vi "Init Robot.vi"(0 "Brake 35":bool=TRUE, 1 "Brake 40":bool=TRUE, 4 "Brake Switch 40":bool=TRUE, 5 "Brake Switch 35":bool=TRUE, 6 "Left Pot Gradient":dbl, 7 "Right Pot Gradient":dbl, 8 "Left Pot Offset":dbl, 9 "Right Pot Offset":dbl) -> (12 "Left Pot Init Reading":dbl, 13 "Right Pot Init Reading":dbl, 14 "Force bias LX":dbl, 15 "Force bias LY":dbl, 16 "Force bias RX":dbl, 17 "Force bias RY":dbl, 18 "Initial Translation":dbl, 19 "Initial Rotation":dbl)   [LabVIEW 2019]
uses:
  <vilib>/myRIO/Instrument Drivers/Onboard IO/AO/typedefs/AO Reference.ctl
  <vilib>/myRIO/Common/Instrument Driver Framework/Utilities/typedefs/myRIO Generic Hardware Reference.ctl
  <vilib>/myRIO/Common/Instrument Driver Framework/Utilities/typedefs/Hardware Version Enum.ctl
  <vilib>/myRIO/Common/Instrument Driver Framework/Utilities/typedefs/myRIO v1.0 Reference.ctl
  <vilib>/myRIO/Common/Instrument Driver Framework/Utilities/typedefs/Generic FPGA Reference.ctl
  <vilib>/myRIO/Common/Instrument Driver Framework/myRIO v1.0/AO/typedefs/AO Channels List.ctl
  <vilib>/myRIO/Common/Instrument Driver Framework/myRIO v1.0/AO/typedefs/AO Channels Enum.ctl
  <vilib>/myRIO/Common/Instrument Driver Framework/Utilities/typedefs/Analog Scaling Constants List.ctl
  <vilib>/myRIO/Common/Instrument Driver Framework/Utilities/typedefs/Analog Scaling Constants.ctl
  <vilib>/userDefined/High Color/nirio_resource_hc.ctl
  <vilib>/myRIO/Instrument Drivers/Onboard IO/DIO/typedefs/DIO Reference.ctl
  <vilib>/myRIO/Common/Instrument Driver Framework/myRIO v1.0/DIO/typedefs/DIO Channels List.ctl
  <vilib>/myRIO/Common/Instrument Driver Framework/myRIO v1.0/DIO/typedefs/DIO Channels Enum.ctl
  <vilib>/myRIO/Instrument Drivers/Onboard IO/AI/typedefs/AI Reference.ctl
  <vilib>/myRIO/Common/Instrument Driver Framework/myRIO v1.0/AI/typedefs/AI Channels List.ctl
  <vilib>/myRIO/Common/Instrument Driver Framework/myRIO v1.0/AI/typedefs/AI Channels Enum.ctl
  <vilib>/myRIO/Common/Instrument Driver Framework/myRIO v1.0/Encoder/typedefs/Encoder Signal Mode.ctl
  <vilib>/myRIO/Instrument Drivers/Onboard IO/Encoder/typedefs/Encoder Reference.ctl
  <vilib>/myRIO/Common/Instrument Driver Framework/myRIO v1.0/Encoder/typedefs/Encoder Channels Enum.ctl
  <vilib>/myRIO/Common/Instrument Driver Framework/myRIO v1.0/Encoder/typedefs/Encoder Configuration v1.0.ctl
  <vilib>/myRIO/Common/Instrument Driver Framework/Utilities/vis/Is FPGA Ref Available.vi
  <vilib>/myRIO/Common/Instrument Driver Framework/myRIO v1.0/AO/vis/myRIO v1.1 Open AO.vi
  <vilib>/myRIO/Instrument Drivers/Onboard IO/AO/vis/Write.vi
  <vilib>/myRIO/Common/Instrument Driver Framework/myRIO v1.0/DIO/vis/myRIO v1.1 Open DIO.vi
  <vilib>/myRIO/Instrument Drivers/Onboard IO/DIO/vis/Write.vi
  <vilib>/myRIO/Common/Instrument Driver Framework/myRIO v1.0/AI/vis/myRIO v1.1 Open AI.vi
  <vilib>/myRIO/Instrument Drivers/Onboard IO/AI/vis/Read.vi
  <vilib>/myRIO/Common/Instrument Driver Framework/myRIO v1.0/Encoder/vis/myRIO v1.1 Open Encoder.vi
  <vilib>/myRIO/Instrument Drivers/Onboard IO/Encoder/vis/Read.vi
  <vilib>/myRIO/Common/Instrument Driver Framework/Utilities/vis/Validate Channels.vi
  <vilib>/myRIO/Common/Instrument Driver Framework/myRIO v1.0/AO/vis/myRIO v1.0 Reserve AO.vi
  <vilib>/myRIO/Common/Instrument Driver Framework/myRIO v1.0/DIO/vis/myRIO v1.0 Reserve DIO.vi
  <vilib>/myRIO/Common/Instrument Driver Framework/myRIO v1.0/AI/vis/myRIO v1.0 Reserve AI.vi
  <vilib>/myRIO/Common/Instrument Driver Framework/myRIO v1.0/Encoder/vis/myRIO v1.0 Reserve Encoder.vi
  <vilib>/myRIO/Common/Instrument Driver Framework/myRIO v1.0/AO/vis/myRIO v1.0 Build MUX Configuration AO.vi
  <vilib>/myRIO/Common/Instrument Driver Framework/myRIO v1.0/Resource Manager/vis/myRIO v1.0 Reserve Channel List.vi
  <vilib>/myRIO/Common/Instrument Driver Framework/myRIO v1.0/DIO/vis/myRIO v1.0 Build MUX Configuration DIO.vi
  <vilib>/myRIO/Common/Instrument Driver Framework/myRIO v1.0/AI/vis/myRIO v1.0 Build MUX Configuration AI.vi
  <vilib>/myRIO/Common/Instrument Driver Framework/myRIO v1.0/Encoder/vis/myRIO v1.0 Build MUX Configuration Encoder.vi
  <vilib>/myRIO/Common/Instrument Driver Framework/myRIO v1.0/Resource Manager/vis/myRIO v1.0 Reserve Channel.vi
  <vilib>/myRIO/Common/Instrument Driver Framework/myRIO v1.0/Resource Manager/vis/myRIO v1.0 Unreserve Channel.vi
  <vilib>/myRIO/Common/Instrument Driver Framework/myRIO v1.0/Resource Manager/vis/myRIO v1.0 Create Configuration List.vi
  <vilib>/myRIO/Common/Instrument Driver Framework/myRIO v1.0/Resource Manager/vis/myRIO v1.0 Build Mutex Name.vi
  <vilib>/Utility/VariantDataType/GetNumericInfo.vi
  <vilib>/Utility/error.llb/Error Cluster From Error Code.vi
  <vilib>/myRIO/Common/Instrument Driver Framework/myRIO v1.0/myRIO v1.1 Open.vi
  <vilib>/myRIO/Common/Instrument Driver Framework/myRIO v1.0/AO/vis/myRIO v1.0 Get Scaling Constants AO.vi
  <vilib>/myRIO/Common/Instrument Driver Framework/Utilities/vis/IO Manager.vi
  <vilib>/myRIO/Common/Instrument Driver Framework/Utilities/vis/Configuration Manager.vi
  <vilib>/myRIO/Common/Instrument Driver Framework/myRIO v1.0/myRIO v1.0 Close.vi
  <vilib>/myRIO/Common/Instrument Driver Framework/myRIO v1.0/AO/vis/myRIO v1.0 Write AO.vi
  <vilib>/myRIO/Common/Instrument Driver Framework/myRIO v1.0/Resource Manager/vis/myRIO v1.0 Configure IO.vi
  <vilib>/myRIO/Common/Instrument Driver Framework/myRIO v1.0/DIO/vis/myRIO v1.0 Write DIO.vi
  <vilib>/myRIO/Common/Instrument Driver Framework/myRIO v1.0/AI/vis/myRIO v1.0 Get Scaling Constants AI.vi
  <vilib>/myRIO/Common/Instrument Driver Framework/myRIO v1.0/AI/vis/myRIO v1.0 Read AI.vi
  <vilib>/myRIO/Common/Instrument Driver Framework/myRIO v1.0/Encoder/vis/myRIO v1.0 Configure Encoder.vi
  <vilib>/myRIO/Common/Instrument Driver Framework/myRIO v1.0/Encoder/vis/myRIO v1.0 Read Encoder.vi
  <vilib>/myRIO/Express VI/Onboard IO/AO/AO Express VI.xnode
  <vilib>/myRIO/Instrument Drivers/Onboard IO/AO/vis/myRIO AO Open.xnode
  <vilib>/myRIO/Express VI/Onboard IO/DO/DO Express VI.xnode
  <vilib>/myRIO/Instrument Drivers/Onboard IO/DIO/vis/myRIO DIO Open.xnode
  <vilib>/myRIO/Express VI/Onboard IO/AI/AI Express VI.xnode
  <vilib>/myRIO/Instrument Drivers/Onboard IO/AI/vis/myRIO AI Open.xnode
  <vilib>/myRIO/Express VI/Onboard IO/Encoder/Encoder Express VI.xnode
  <vilib>/myRIO/Instrument Drivers/Onboard IO/Encoder/vis/myRIO Encoder Open.xnode
  <vilib>/myRIO/Common/Instrument Driver Framework/myRIO v1.0/Encoder/typedefs/Encoder Count Direction Enum.ctl
  <vilib>/myRIO/Instrument Drivers/Onboard IO/Encoder/Encoder.lvlib
  <vilib>/myRIO/Instrument Drivers/Onboard IO/DIO/DIO.lvlib
  <vilib>/myRIO/Instrument Drivers/Onboard IO/AO/AO.lvlib
  <vilib>/myRIO/Instrument Drivers/Onboard IO/AI/AI.lvlib
panel:
  out "VoltageTranslation":dbl
  out "VoltageRotation":dbl
  out "Encoder Counter Value":i32(graph)
  out "Encoder Counter Value 2":i32(graph)
  out "P Rotation":dbl
  out "P Translation":dbl
  out "left init":dbl
  out "right init":dbl
  out "Rot Pot":dbl
  # "This Vi starts all task, calculates the initals values of all sensores and encoder and can open the brakes if needed."
  # "Output:"
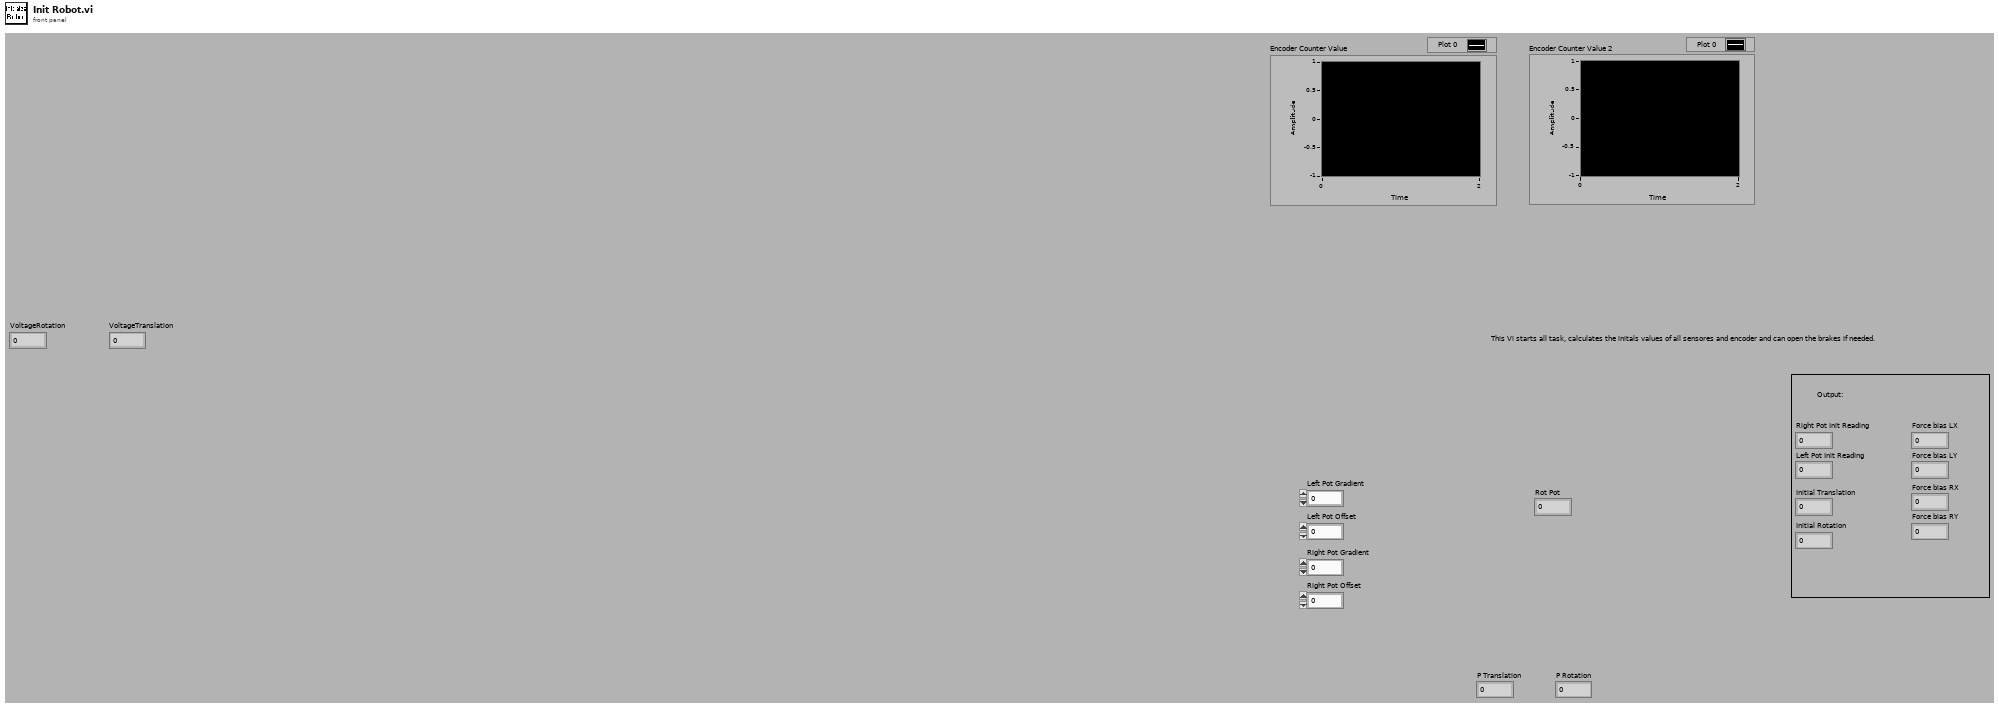
[diagram p1: front panel]
types:
  T1 = typedef "AO.lvlib/AO Reference.ctl" = cluster{"myRIO Reference":T2, "AO Channel List":T6, "AO Scaling Constant List":T8}
  T2 = typedef "myRIO Generic Hardware Reference.ctl" = cluster{"myRIO Model":T3, "myRIO Hardware Reference":T4}
  T3 = typedef "Hardware Version Enum.ctl" = enum16{"Unknown", "myRIO-1900", "myRIO-1950", "roboRIO", "NI ELVIS RIO CM", "ELVIS III"}
  T4 = typedef "myRIO v1.0 Reference.ctl" = cluster{"Generic FPGA Reference":T5, "Allow multiple opens":bool}
  T5 = typedef "Generic FPGA Reference.ctl" = refnum<k20>
  T6 = typedef "AO Channels List.ctl" = T7[]
  T7 = typedef "AO Channels Enum.ctl" = enum16{"Not Connected", "AudioOut/Left", "AudioOut/Right", "C/AO0", "C/AO1", "A/AO0", "A/AO1", "B/AO0", "B/AO1"}
  T8 = typedef "Analog Scaling Constants List.ctl" = T9[]
  T9 = typedef "Analog Scaling Constants.ctl" = cluster{"LSB Weight (Volts)":dbl, "Offset (Volts)":dbl, "Signed?":bool}
  T10 = typedef "nirio_resource_hc.ctl" = tag
  T11 = typedef "DIO.lvlib/DIO Reference.ctl" = cluster{"myRIO Reference":T2, "DIO Channels List":T12}
  T12 = typedef "DIO Channels List.ctl" = T13[]
  T13 = typedef "DIO Channels Enum.ctl" = enum16{"Not Connected", "C/DIO0", "C/DIO1", "C/DIO2", "C/DIO3", "C/DIO4", "C/DIO5", "C/DIO6", "C/DIO7", "A/DIO0", "A/DIO1", "A/DIO2", "A/DIO3", "A/DIO4", "A/DIO5", "A/DIO6", "A/DIO7", "A/DIO8", "A/DIO9", "A/DIO10", "A/DIO11", "A/DIO12", "A/DIO13", "A/DIO14", "A/DIO15", "A/DIO16", "A/DIO17", "A/DIO18", "A/DIO19", "B/DIO0", "B/DIO1", "B/DIO2", "B/DIO3", "B/DIO4", "B/DIO5", "B/DIO6", "B/DIO7", "B/DIO8", "B/DIO9", "B/DIO10", "B/DIO11", "B/DIO12", "B/DIO13", "B/DIO14", "B/DIO15", "B/DIO16", "B/DIO17", "B/DIO18", "B/DIO19", "LED0", "LED1", "LED2", "LED3", "Button0", "DIO/DIO0", "DIO/DIO1", "DIO/DIO2", "DIO/DIO3", "DIO/DIO4", "DIO/DIO5", "DIO/DIO6", "DIO/DIO7", "DIO/DIO8", "DIO/DIO9", "SPI/CS0", "SPI/CS1", "SPI/CS2", "SPI/CS3", "LED RADIO (Green)", "LED RADIO (Red)", "LED COMM (Green)", "LED COMM (Red)", "LED MODE (Green)", "LED MODE (Red)"}
  T14 = typedef "AI.lvlib/AI Reference.ctl" = cluster{"myRIO Reference":T2, "AI Channels List":T15, "AI Scaling Constants List":T8}
  T15 = typedef "AI Channels List.ctl" = T16[]
  T16 = typedef "AI Channels Enum.ctl" = enum16{"Not Connected", "AudioIn/Left", "AudioIn/Right", "C/AI0", "C/AI1", "A/AI0", "A/AI1", "A/AI2", "A/AI3", "A/AI4", "A/AI5", "A/AI6", "A/AI7", "B/AI0", "B/AI1", "B/AI2", "B/AI3", "B/AI4", "B/AI5", "B/AI6", "B/AI7", "AI/AI0", "AI/AI1", "AI/AI2", "AI/AI3", "A/AI0 (DIFF)", "A/AI1 (DIFF)", "A/AI2 (DIFF)", "A/AI3 (DIFF)", "B/AI0 (DIFF)", "B/AI1 (DIFF)", "B/AI2 (DIFF)", "B/AI3 (DIFF)"}
  T17 = typedef "Encoder.lvlib/Encoder Reference.ctl" = cluster{"myRIO Reference":T2, "Encoder Channels Enum":T18}
  T18 = typedef "Encoder Channels Enum.ctl" = enum16{"Not Connected", "C/ENC0", "C/ENC1", "A/ENC", "A/ENC0", "A/ENC1", "A/ENC2", "A/ENC3", "A/ENC4", "A/ENC5", "A/ENC6", "A/ENC7", "A/ENC8", "A/ENC9", "B/ENC", "B/ENC0", "B/ENC1", "B/ENC2", "B/ENC3", "B/ENC4", "B/ENC5", "B/ENC6", "B/ENC7", "B/ENC8", "B/ENC9", "DIO/ENC0", "DIO/ENC1", "DIO/ENC2", "DIO/ENC3", "DIO/ENC4"}
  T19 = typedef "Encoder Signal Mode.ctl" = enum16{"Quadrature phase signal", "Step and direction signal"}
  T20 = cluster{"[0]":dbl, "[1]":dbl, "[2]":dbl, "[3]":dbl, "[4]":dbl, "[5]":dbl, "[6]":dbl, "[7]":dbl, "[8]":dbl}
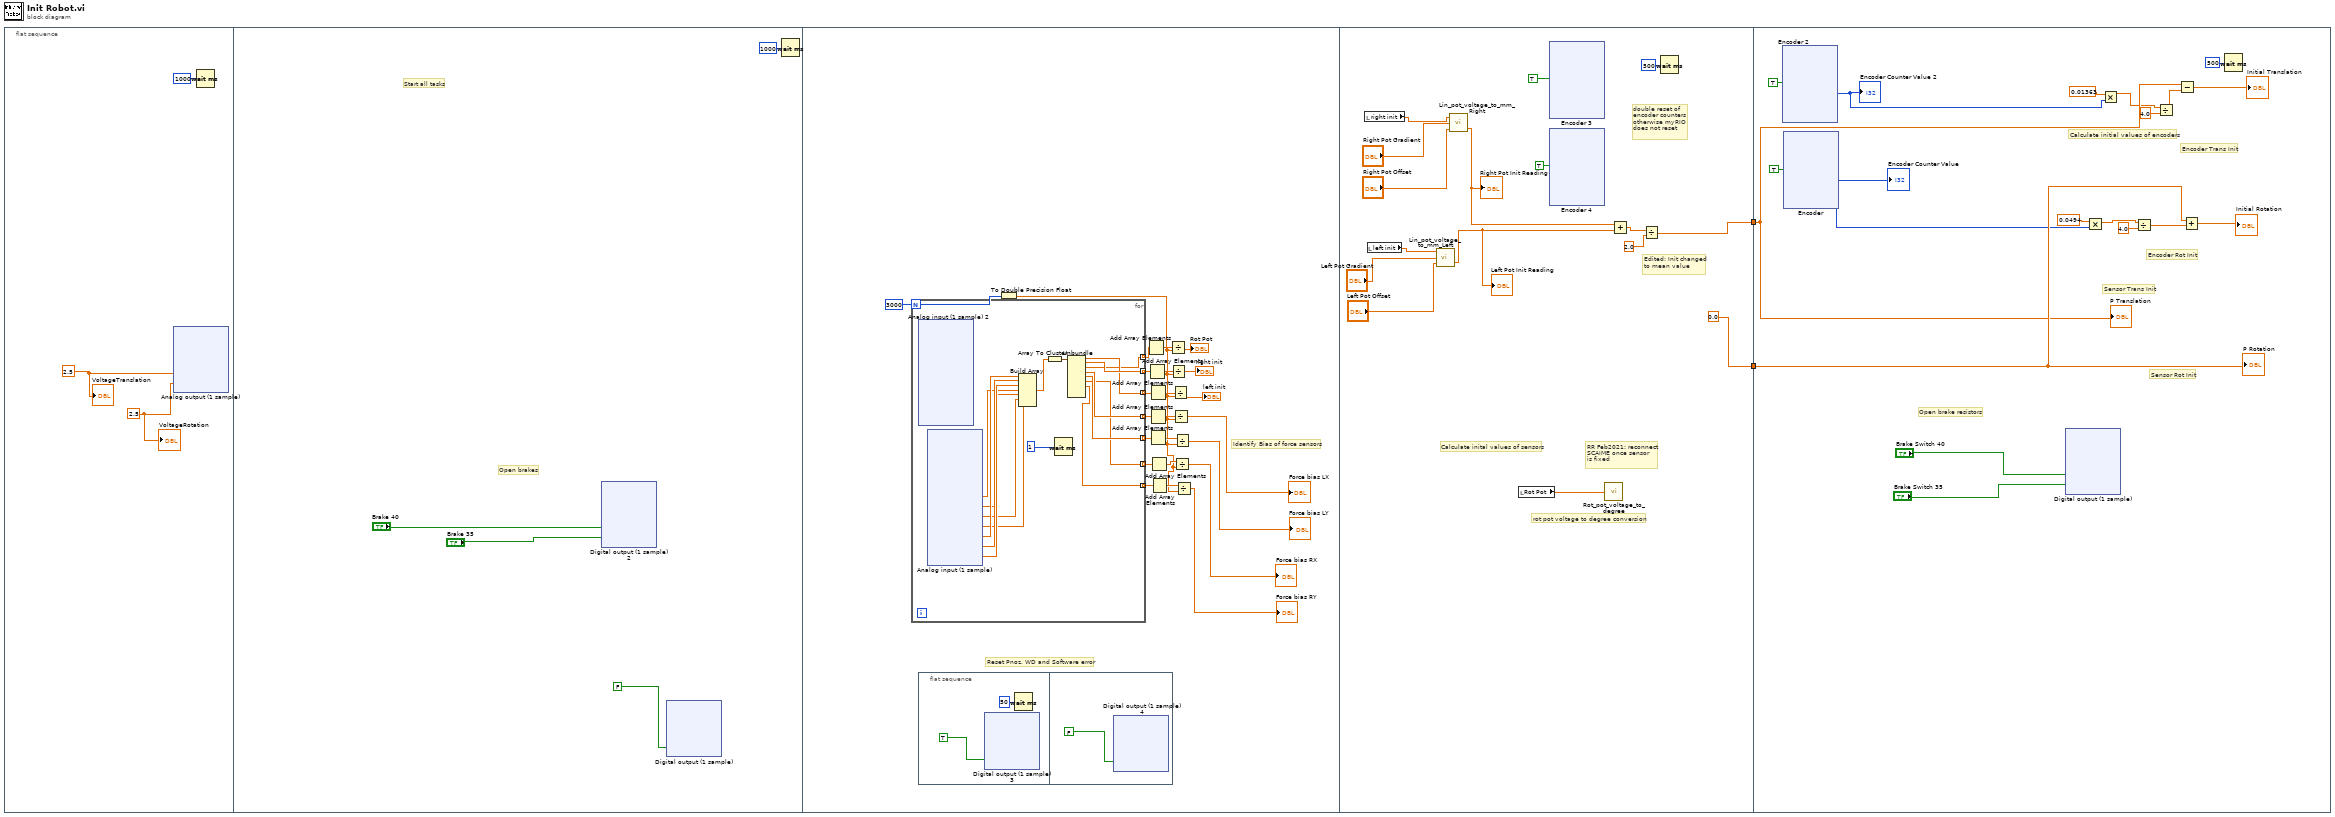
[diagram p0: block diagram]
diagram:
  n1 = flat-sequence {
    tunnel: [w324] -> w2
    tunnel: [0.0] -> w1
    tunnel: w2 -> [w437]
    tunnel: w1 -> [w438]
    frame #0 {
      w3 = 2.5
      w4 = 2.5
      n2 = xnode "Analog output (1 sample)"("Motor1Current_AREAD (B/AO0 (Pin 2))"=w4, "Motor2Current_AREAD (A/AO0 (Pin 2))"=w3) -> ()  [unwired: 1 in, 1 out]
      n3 = Wait (ms)(milliseconds to wait=u32 1000) -> ()  [unwired: 1 out]
      "VoltageRotation" <- w3
      "VoltageTranslation" <- w4
    }
    frame #1 {
      # "Open brakes"
      # "Start all tasks"
      n4 = xnode "Digital output (1 sample) 2"("SIG_REL3 (B/DIO2 (Pin 15))"="Brake 40", "SIG_REL5 (B/DIO4 (Pin 19))"="Brake 35") -> ()  [unwired: 1 in, 1 out]
      n5 = xnode "Digital output (1 sample)"("Safety PILZ (B/DIO0 (Pin 11))"=FALSE ("data")) -> ()  [unwired: 1 in, 1 out]
      n6 = Wait (ms)(milliseconds to wait=u32 1000) -> ()  [unwired: 1 out]
    }
    frame #2 {
      w133 = 3000
      # "Identify Bias of force sensors"
      # "Reset Pnoz, WD and Software error"
      n7 = for {
        N: w133 -> [_]
        tunnel: [w151] -> w138 mode=indexing
        tunnel: [w157] -> w137 mode=indexing
        tunnel: [w152] -> w136 mode=indexing
        tunnel: [w154] -> w129 mode=indexing
        tunnel: [w153] -> w128 mode=indexing
        tunnel: [w147] -> w124 mode=indexing
        tunnel: [w146] -> w123 mode=indexing
        n8 = xnode "Analog input (1 sample) 2"() -> ()  [unwired: 1 in, 6 out]
        n9 = xnode "Analog input (1 sample)"() -> ("ForceSensor_READ1 (C/AI0 (AI0))"=w143:dbl, "ForceSensor_READ2 (C/AI1 (AI1))"=w142:dbl, "ForceSensor_READ3 (B/AI0 (Pin 3))"=w145:dbl, "ForceSensor_READ4 (B/AI1 (Pin 5))"=w144:dbl, "AI_lin_pot_left (A/AI0 (Pin 3))"=w150:dbl, "AI_lin_pot_right (A/AI1 (Pin 5))"=w149:dbl, "AI_rot_pot (A/AI2 (Pin 7))"=w148:dbl)  [unwired: 1 in, 1 out]
        n10 = Build Array(w150, w149, w148, w143, w142, w145, w144) -> (w155:dbl[])
        n11 = Array To Cluster(array=w155) -> (cluster=w158:T20)
        n12 = Wait (ms)(milliseconds to wait=1) -> ()  [unwired: 1 out]
        n13 = Unbundle(w158) -> ("[0]"=w152:dbl, "[1]"=w157:dbl, "[2]"=w151:dbl, "[3]"=w154:dbl, "[4]"=w153:dbl, "[5]"=w147:dbl, "[6]"=w146:dbl)  [unwired: 2 out]
      }
      n14 = flat-sequence {
        frame #0 {
          n15 = xnode "Digital output (1 sample) 3"("Safety PILZ (B/DIO0 (Pin 11))"=TRUE ("data")) -> ()  [unwired: 1 in, 1 out]
          n16 = Wait (ms)(milliseconds to wait=u32 50) -> ()  [unwired: 1 out]
        }
        frame #1 {
          n17 = xnode "Digital output (1 sample) 4"("Safety PILZ (B/DIO0 (Pin 11))"=FALSE ("data")) -> ()  [unwired: 1 in, 1 out]
        }
      }
      n18 = To Double Precision Float(number=w133) -> (double precision float=w125:dbl)
      n19 = Add Array Elements(numeric array=w138) -> (sum=w141:dbl)
      n20 = Add Array Elements(numeric array=w137) -> (sum=w140:dbl)
      n21 = Add Array Elements(numeric array=w129) -> (sum=w131:dbl)
      n22 = Add Array Elements(numeric array=w136) -> (sum=w139:dbl)
      n23 = Add Array Elements(numeric array=w128) -> (sum=w130:dbl)
      n24 = Add Array Elements(numeric array=w124) -> (sum=w126:dbl)
      n25 = Add Array Elements(numeric array=w123) -> (sum=w127:dbl)
      n26 = Divide(x=w141, y=w125) -> (x/y=→"Rot Pot":dbl)
      n27 = Divide(x=w140, y=w125) -> (x/y=→"right init":dbl)
      n28 = Divide(x=w139, y=w125) -> (x/y=→"left init":dbl)
      n29 = Divide(x=w131, y=w125) -> (x/y=→"Force bias LX":dbl)
      n30 = Divide(x=w126, y=w125) -> (x/y=→"Force bias RX":dbl)
      n31 = Divide(x=w130, y=w125) -> (x/y=→"Force bias LY":dbl)
      n32 = Divide(x=w127, y=w125) -> (x/y=→"Force bias RY":dbl)
    }
    frame #3 {
      # "Edited: Init changed to mean value"
      # "rot pot voltage to degree conversion"
      # "RR Feb2021: reconnect\nSCAIME once sensor\nis fixed"
      # "double reset of\nencoder counters\notherwise myRIO\ndoes not reset"
      # "Calculate inital values of sensors"
      n33 = local read "right init"() -> (w323:dbl)
      n34 = local read "left init"() -> (w322:dbl)
      n35 = call "Lin_pot_voltage_to_mm_Left.vi"("Offset"="Left Pot Offset", "Gradient"="Left Pot Gradient", "LinPot Voltage"=w322) -> ("LinPot mm (center to finger)"=w321:dbl)  [unwired: 1 out]
      "Left Pot Init Reading" <- w321
      n36 = call "Lin_pot_voltage_to_mm_Right.vi"("Offset"="Right Pot Offset", "Gradient"="Right Pot Gradient", "LinPot Voltage"=w323) -> ("LinPot mm (center to finger)"=w320:dbl)  [unwired: 1 out]
      "Right Pot Init Reading" <- w320
      n37 = local read "Rot Pot"() -> (w328:dbl)
      n38 = xnode "Encoder 3"("Reset Counter"=TRUE) -> ()  [unwired: 1 in, 4 out]
      n39 = xnode "Encoder 4"("Reset Counter"=TRUE) -> ()  [unwired: 1 in, 4 out]
      n40 = call "Rot_pot_voltage_to_degree.vi"("RotaryPot (Voltage)"=w328) -> ()  [unwired: 1 out]
      n41 = Add(x=w320, y=w321) -> (x+y=w326:dbl)
      n42 = Divide(x=w326, y=2.0) -> (x/y=w324:dbl)
      n43 = Wait (ms)(milliseconds to wait=u32 500) -> ()  [unwired: 1 out]
    }
    frame #4 {
      # "Calculate initial values of encoders"
      # "Open brake resistors"
      # "Encoder Trans Init"
      # "Encoder Rot Init"
      # "Sensor Trans Init"
      # "Sensor Rot Init"
      n44 = xnode "Encoder 2"("Reset Counter"=TRUE) -> ("Counter Value"=w436:i32)  [unwired: 1 in, 3 out]
      "Encoder Counter Value 2" <- w436
      n45 = xnode "Encoder"("Reset Counter"=TRUE) -> ("Counter Value"=w435:i32)  [unwired: 1 in, 3 out]
      "Encoder Counter Value" <- w435
      n46 = xnode "Digital output (1 sample)"("SIG_REL2 (B/DIO1 (Pin 13))"="Brake Switch 40", "SIG_REL4 (B/DIO3 (Pin 17))"="Brake Switch 35") -> ()  [unwired: 1 in, 1 out]
      n47 = Multiply(x=0.0494, y=w435) -> (x*y=w428:dbl)
      n48 = Multiply(x=0.01363, y=w436) -> (x*y=w425:dbl)
      n49 = Divide(x=w428, y=4.0) -> (x/y=w427:dbl)
      n50 = Divide(x=w425, y=4.0) -> (x/y=w424:dbl)
      n51 = Subtract(x=w437, y=w424) -> (x-y=→"Initial Translation":dbl)
      n52 = Add(x=w438, y=w427) -> (x+y=→"Initial Rotation":dbl)
      n53 = Wait (ms)(milliseconds to wait=u32 500) -> ()  [unwired: 1 out]
      "P Translation" <- w437
      "P Rotation" <- w438
    }
  }
